vi "Analog Set Reference Voltage.vi"(8 "Error In":errorcluster={"status"=TRUE, "code"=5001, "source"="LVH-LINX.lvlib:Generate Error.vi<ERR>\nA timeout occured while waiting for the LINX device to respond."}, 9 "Voltage (V)":dbl, 10 "Analog Reference Mode":T1, 11 "LINX Device Config":T2={"Interface"=enum."Serial", "COM Port"="COM5", "TCP Configuration"={"IP Address"="", "Port"=0}, "Device Family"=0, "Device ID"=0, "Device Name"="", "TCP Ref"=refnum, "Channels"={"DI"=[], "DO"=[], "AI"=[], "AO"=[], "PWM"=[], "QE"=[], "UART"=[], "I2C 2"=[], "SPI"=[], "CAN"=[], "Servo"=[], "AI Ref (V)"=0.0, "AO Ref (V)"=0.0, "AO Resolution (Bits)"=0}}) -> (0 "Error Out":errorcluster={"status"=TRUE, "code"=5001, "source"="LVH-LINX.lvlib:Generate Error.vi<ERR>\nA timeout occured while waiting for the LINX device to respond."}, 3 "LINX Device Config":T2={"Interface"=enum."Serial", "COM Port"="COM5", "TCP Configuration"={"IP Address"="", "Port"=0}, "Device Family"=0, "Device ID"=0, "Device Name"="", "TCP Ref"=refnum, "Channels"={"DI"=[], "DO"=[], "AI"=[], "AO"=[], "PWM"=[], "QE"=[], "UART"=[], "I2C 2"=[], "SPI"=[], "CAN"=[], "Servo"=[], "AI Ref (V)"=0.0, "AO Ref (V)"=0.0, "AO Resolution (Bits)"=0}})   [LabVIEW 2011, in "LMH-LINX.lvlib" / "Device.lvlib"]
uses:
  Device.lvlib
  Type Defs/LINX Device Config.ctl
  Type Defs/Interface.ctl
  Type Defs/TCP Config.ctl
  Type Defs/Channels.ctl
  Type Defs/AI Reference Mode.ctl
  Type Defs/Error Type.ctl
  LMH-LINX.lvlib
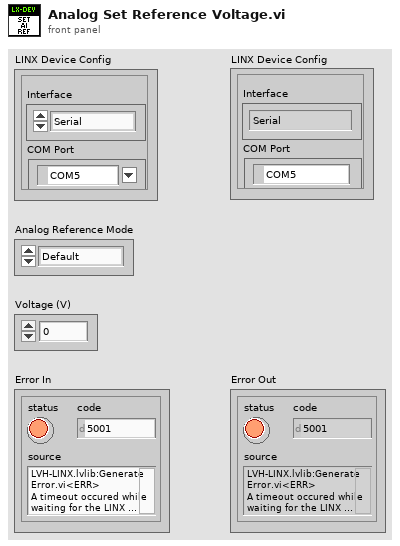
[diagram p1: front panel]
types:
  T1 = typedef "LMH-LINX.lvlib/Device.lvlib/AI Reference Mode.ctl" = enum16{"Default", "Internal", "External"}
  T2 = typedef "LMH-LINX.lvlib/Device.lvlib/LINX Device Config.ctl" = cluster{"Interface":T3, "COM Port":refnum<visa-resource-name>, "TCP Configuration":T4, "Device Family":u8, "Device ID":u8, "Device Name":string, "TCP Ref":refnum<k5>, "Channels":T5}
  T3 = typedef "LMH-LINX.lvlib/Interface.ctl" = enum16{"Serial", "TCP"}
  T4 = typedef "LMH-LINX.lvlib/Device.lvlib/TCP Config.ctl" = cluster{"IP Address":string, "Port":u16}
  T5 = typedef "LMH-LINX.lvlib/Channels.ctl" = cluster{"DI":u8[], "DO":u8[], "AI":u8[], "AO":u8[], "PWM":u8[], "QE":u8[], "UART":u8[], "I2C 2":u8[], "SPI":u8[], "CAN":u8[], "Servo":u8[], "AI Ref (V)":dbl, "AO Ref (V)":dbl, "AO Resolution (Bits)":u8}
  T6 = typedef "LMH-LINX.lvlib/Error Type.ctl" = enum16{"Unknown", "Timeout", "Corrupt Return Packet", "Unable To Connect", "Command Not Supported", "Channel DNE", "Invalid COM Config", "Firmware Version Mismatch", "myRIO Support", "CMD Specific Error"}
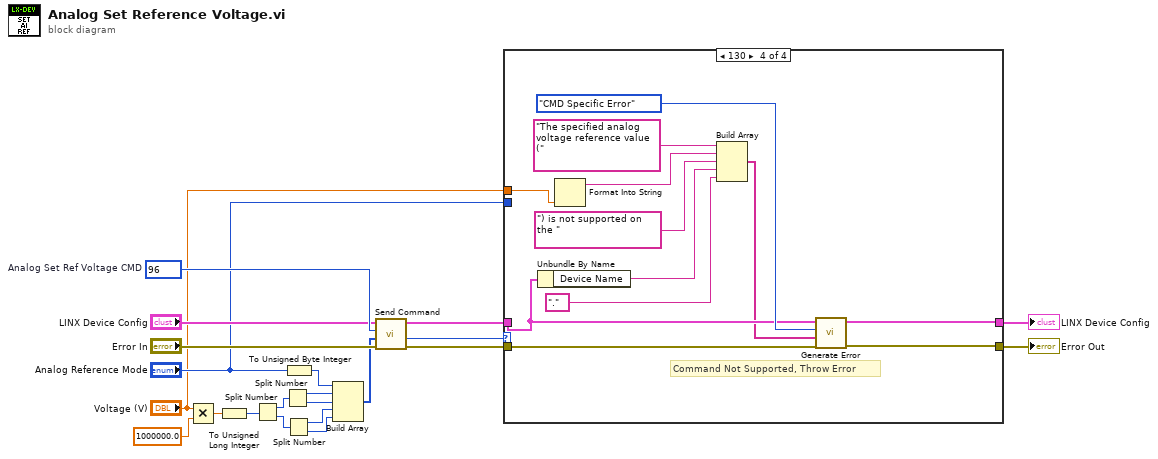
[diagram p0: block diagram]
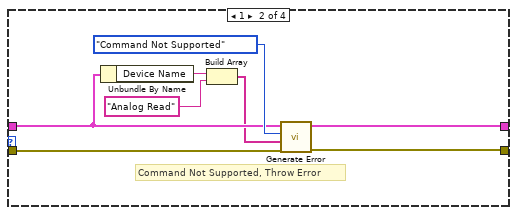
[diagram p3: hidden frame]
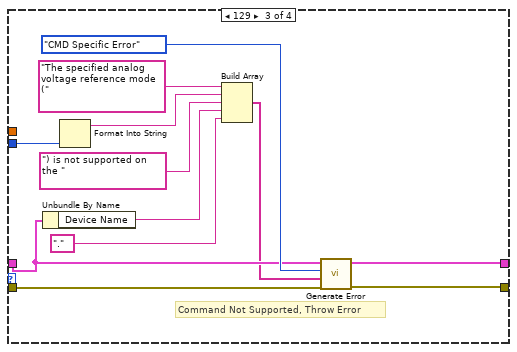
[diagram p4: hidden frame]
diagram:
  w20 = u16 96  # Analog Set Ref Voltage CMD
  n1 = Multiply(x="Voltage (V)", y=1000000.0) -> (x*y=w11:dbl)
  n2 = To Unsigned Long Integer(number=w11) -> (unsigned 32bit integer=w10:u32)
  n3 = Split Number(x=w10) -> (hi(x)=w8:u16, lo(x)=w9:u16)
  n4 = Split Number(x=w8) -> (hi(x)=w7:u8, lo(x)=w6:u8)
  n5 = To Unsigned Byte Integer(number="Analog Reference Mode") -> (unsigned 8bit integer=w13:u8)
  n6 = Split Number(x=w9) -> (hi(x)=w5:u8, lo(x)=w4:u8)
  n7 = Build Array(w13, w7, w6, w5, w4) -> (w3:u8[])
  n8 = call "Send Command.vi"("Error In"="Error In", "ARGS"=w3, "CMD"=w20, "LINX Device Config"="LINX Device Config") -> ("Error Out"=w16:errorcluster, "Status"=w14:u8, "LINX Device Config"=w18:T2)  [unwired: 4 in, 1 out]
  n9 = case shown="130" w14 {
    tunnel: [w22 w29 w41 w53] -> w19
    tunnel: w18 -> [w22 w25 w39 w51]
    tunnel: [w23 w30 w42 w54] -> w17
    tunnel: w16 -> [w23 w31 w43 w55]
    tunnel: "Analog Reference Mode" -> [_ _ w38 _]
    tunnel: "Voltage (V)" -> [_ _ _ w44]
    frame 0, Default {
    }
    frame 1 {
      # "Command Not Supported, Throw Error"
      n10 = Unbundle By Name(w25) -> ("Device Name"=w27:string)
      n11 = Build Array(w27, "Analog Read") -> (w24:string[])
      n12 = call "Generate Error.vi"("Error In"=w31, "Arguments"=w24, "Error Type"=Error_Type."Command Not Supported", "LINX Device Config"=w25) -> ("Error Out"=w30:errorcluster, "LINX Device Config"=w29:T2)  [unwired: 6 in]
    }
    frame 129 {
      # "Command Not Supported, Throw Error"
      n13 = Unbundle By Name(w39) -> ("Device Name"=w34:string)
      n14 = Format Into String(w38) -> (resulting string=w36:string)  [unwired: 3 in, 1 out]
      n15 = Build Array("The specified analog voltage reference mode (", w36, ") is not supported on the ", w34, ".") -> (w32:string[])
      n16 = call "Generate Error.vi"("Error In"=w43, "Arguments"=w32, "Error Type"=Error_Type."CMD Specific Error", "LINX Device Config"=w39) -> ("Error Out"=w42:errorcluster, "LINX Device Config"=w41:T2)  [unwired: 6 in]
    }
    frame 130 {
      # "Command Not Supported, Throw Error"
      n17 = Unbundle By Name(w51) -> ("Device Name"=w47:string)
      n18 = Format Into String(w44) -> (resulting string=w49:string)  [unwired: 3 in, 1 out]
      n19 = Build Array("The specified analog voltage reference value (", w49, ") is not supported on the ", w47, ".") -> (w45:string[])
      n20 = call "Generate Error.vi"("Error In"=w55, "Arguments"=w45, "Error Type"=Error_Type."CMD Specific Error", "LINX Device Config"=w51) -> ("Error Out"=w54:errorcluster, "LINX Device Config"=w53:T2)  [unwired: 6 in]
    }
  }
  "Error Out" <- w17
  "LINX Device Config" <- w19
